vi "SUB_TP_Output.vi"(3 "Measured C":dbl format="%_6f", 4 "SPEC MAX C":dbl format="%#_8f", 5 "SPEC MIN C":dbl format="%_6f", 6 "Test Item":string) -> (0 "Measured Voltage":string, 1 "result":T1, 2 "結果":bool)   [LabVIEW 2011]
panel:
  out "In Range?":bool
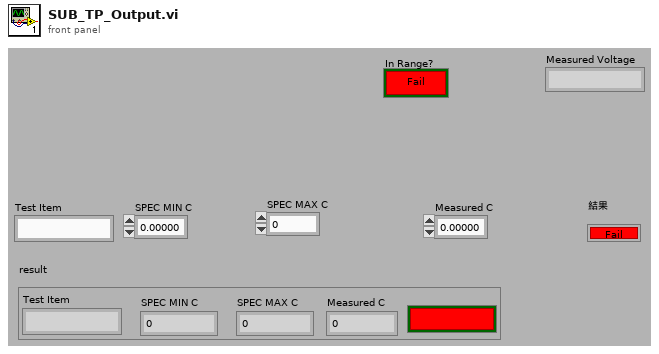
[diagram p1: front panel]
types:
  T1 = cluster{"Test Item":string, "SPEC MIN C":dbl, "SPEC MAX C":dbl, "Measured C":dbl, bool}
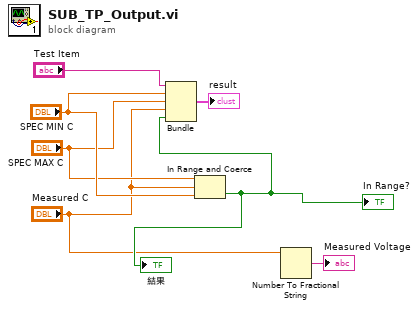
[diagram p0: block diagram]
diagram:
  n1 = In Range and Coerce(upper limit="SPEC MAX C", x="Measured C", lower limit="SPEC MIN C") -> (In Range?=w5:bool)  [unwired: 1 out]
  "結果" <- w5
  "In Range?" <- w5
  n2 = Bundle("Test Item"="Test Item", "SPEC MIN C"="SPEC MIN C", "SPEC MAX C"="SPEC MAX C", "Measured C"="Measured C", w5) -> (→"result":T1)  [unwired: 1 in]
  n3 = Number To Fractional String(number="Measured C") -> (F-format string=→"Measured Voltage":string)  [unwired: 3 in]
